vi "Features_SpecPage.vi"(10 "Spec Page Interface":T5, 11 "MetaDataObj in":refnum<class "MetaDataObj.lvclass">) -> (3 "MetaDataObj out":refnum<class "MetaDataObj.lvclass">)   [LabVIEW 2013, in "FixedChannelTBModuleDecideFeatures.lvclass"]
uses:
  FixedChannelTBModuleDecideFeatures.lvclass
  <resource>/dialog/NewProjectWizard/Spec Page Interface.ctl
  <resource>/dialog/NewProjectWizard/MetaDataObj/MetaDataObj.lvclass
  channel configuration.ctl
  <vilib>/NI/Tag Bus Module Framework/channel/channel classification.ctl
  <vilib>/NI/Tag Bus/tag/Data Type.ctl
  <resource>/dialog/NewProjectWizard/MetaDataObj/MetaDataObj.lvclass/MetaDataObj.ctl
  FixedChannelTBModuleDecideFeatures.lvclass/FixedChannelTBModuleDecideFeatures.ctl
  <resource>/dialog/NewProjectWizard/MetaDataObj/Accessors/Write Project Name.vi
  <resource>/dialog/NewProjectWizard/MetaDataObj/Accessors/Write Project Root.vi
  Write component name.vi
  Write instances allowed.vi
  <resource>/dialog/NewProjectWizard/MetaDataObj/Accessors/Write File Prefix.vi
  <vilib>/NI/Tag Bus Module Framework/channel/TBM channel.lvclass
  <vilib>/NI/Tag Bus/tag/tag descriptor.lvclass
panel:
  in  "Tab Control":T1(tab)
  in  "Channels to create":T2[](array[typedef])
  in  "Instances Allowed":i32=-1
  in  "Module Name":string
  in  "Project Root":path
  # "This script will generate a TBM with three methods in which you can add logic: User Input, User Process, and User Output. Before running this script, specify the Channel Name and Data Type for each element of data that you'd like those methods to interact with. Their are also 4 channel types to choose from.  An input channel is data generated by the input function. A processing parameter is an input to the processing function which returns processing results.  Finally an output channel is data that is passed into the output method.  \n\nThese channels can be modified later by running the User Control Module script from the LabVIEW Tools menu."
  # "Channel Name"
  # "Data Type"
  # "Channel Type"
  # "Execution Behaviors:"
  # "Number of classes allowed in a system. Default is infinite, -1. Examples: {Scaling: -1};{Scan Engine: 1}"
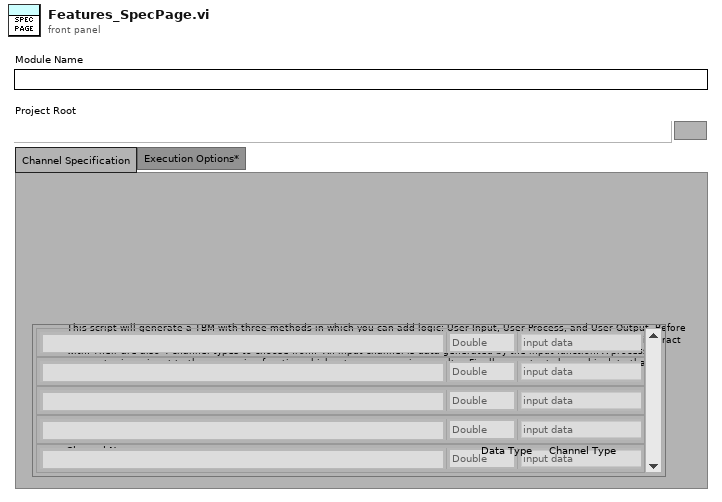
[diagram p1: front panel]
types:
  T1 = enum32{"Channel Specification", "Execution Options*"}
  T2 = typedef "FixedChannelTBModuleDecideFeatures.lvclass/channel configuration.ctl" = cluster{"Name":string, "channel classification":T3, "data type":T4}
  T3 = typedef "TBM channel.lvclass/channel classification.ctl" = enum16{"input data", "output data", "processing parameter", "processing result"}
  T4 = typedef "tag bus.lvlib/tag descriptor.lvclass/Data Type.ctl" = enum16{"Double", "Single", "I64", "I32", "I16", "I8", "U64", "U32", "U16", "U8", "Boolean", "String", "Array of Double", "Array of Single", "Array of I64", "Array of I32", "Array of I16", "Array of I8", "Array of U64", "Array of U32", "Array of U16", "Array of U8", "Array of Boolean", "Array of String"}
  T5 = typedef "Spec Page Interface.ctl" = cluster{"\"Tab Forward To\" Refnum":refnum<vi>, "\"Tab Backward To\" Refnum":refnum<vi>, "Errors":refnum<user-event>, "Quit":refnum<user-event>}
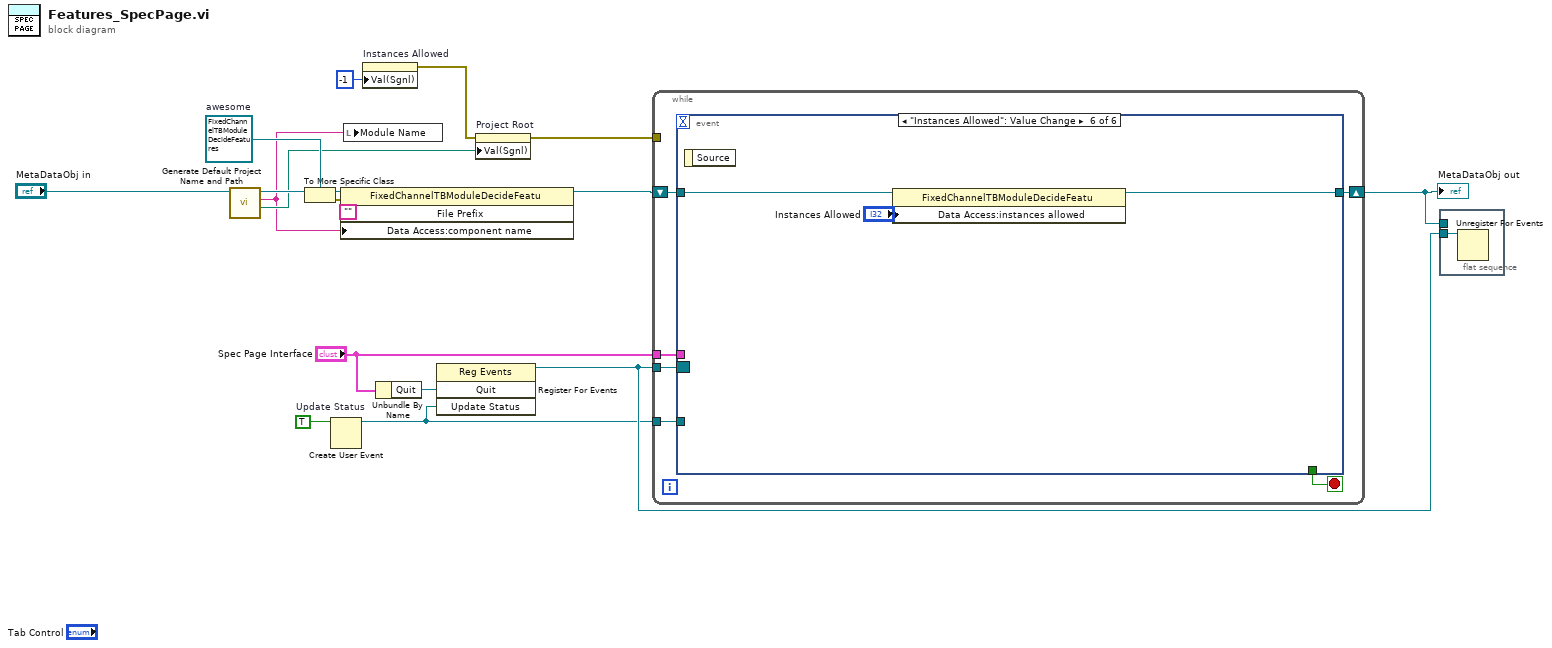
[diagram p0: block diagram]
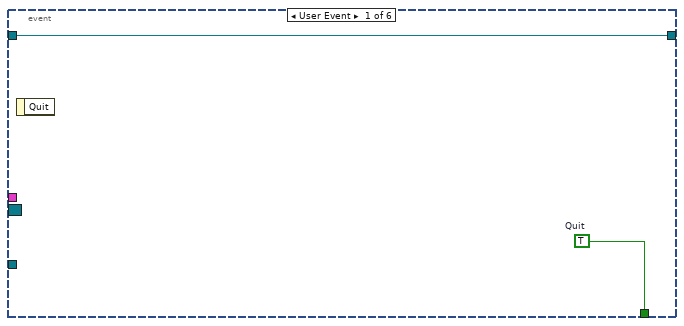
[diagram p2: hidden frame]
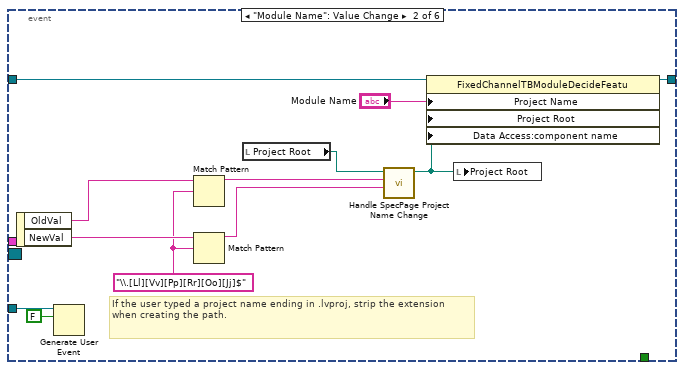
[diagram p3: hidden frame]
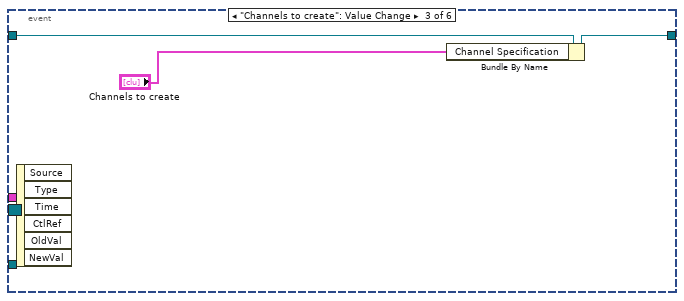
[diagram p4: hidden frame]
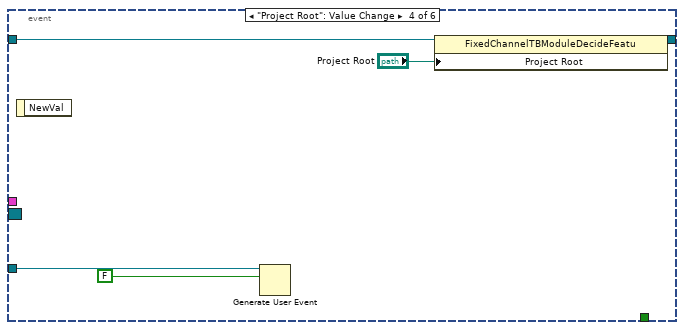
[diagram p5: hidden frame]
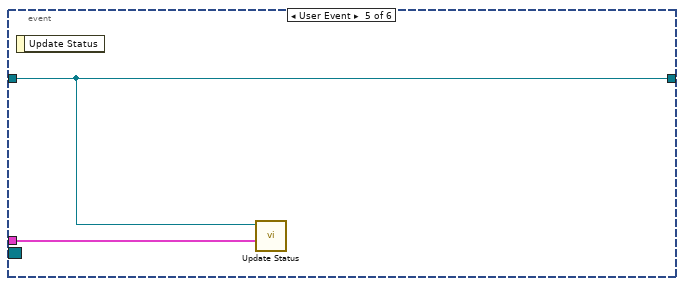
[diagram p6: hidden frame]
diagram:
  w12 = TRUE  # Update Status
  w13 = refnum<class "FixedChannelTBModuleDecideFeatures.lvclass"> refnum  # awesome
  n1 = call <resource>:"Generate Default Project Name and Path.vi"("DNL_MetaDataObj in"="MetaDataObj in") -> ("Project Root"=w5:path, "Project Name"=w3:string, "DNL_MetaDataObj out"=w6:refnum<class "MetaDataObj.lvclass">)  [unwired: 8 in]
  n2 = To More Specific Class(target class=w13, reference=w6) -> (specific class reference=w15:refnum<class "FixedChannelTBModuleDecideFeatures.lvclass">, error out=w14:errorcluster)  [unwired: 1 in]
  n3 = Create User Event(user event datatype=w12) -> (user event=w9:refnum<user-event>)  [unwired: 1 in, 1 out]
  n4 = property class="FixedChannelTBModuleDecideFeatu"(reference=w15, error in=w14, "File Prefix"="", "Data Access:component name"=w3) -> (reference out=w11:refnum<class "FixedChannelTBModuleDecideFeatures.lvclass">)  [unwired: 1 out]
  n5 = local write "Module Name"(w3) -> ()
  n6 = property on="Instances Allowed" class="DigNum (strict)"("Val(Sgnl)"=-1 ("Value (Signaling)")) -> (error out=w2:errorcluster)  [unwired: 2 in, 1 out]
  n7 = Unbundle By Name("Spec Page Interface") -> ("Quit"=w18:refnum<user-event>)
  n8 = register-events(w18, w9) -> (reference out=w17:refnum<event-registration>)  [unwired: 2 in, 1 out]
  n9 = property on="Project Root" class="Path"(error in=w2, "Val(Sgnl)"=w5) -> (error out=w10:errorcluster)  [unwired: 1 in, 1 out]
  n10 = while {
    tunnel: "Spec Page Interface" -> [w23]
    shift-right: [w21] -> w4
    shift-left: w11 -> [w20]
    tunnel: w17 -> [w22]
    tunnel: w10 -> [_]
    tunnel: w9 -> [w19]
    stop <- w24 stop-if-true
    n11 = event shown="[5] \"Instances Allowed\": Value Change" {
      selector: w22 -> [_ _ _ _ _ _]
      dyn-events: _ -> [_ _ _ _ _ _]
      timeout: _ -> [_ _ _ _ _ _]
      tunnel: w23 -> [_ _ _ _ w47 _]
      tunnel: [w26 _ _ _ _ _] -> w24
      tunnel: [w25 w38 w40 w45 w48 w50] -> w21
      tunnel: w20 -> [w25 w35 w41 w46 w48 w51]
      tunnel: w19 -> [_ w37 _ w44 _ _]
      event User Event {
        w26 = TRUE  # Quit
        n12 = event-data() -> ()  [unwired: 1 in, 1 out]
      }
      event "Module Name": Value Change {
        w30 = "\\.[Ll][Vv][Pp][Rr][Oo][Jj]$" ("regular expression")
        # "If the user typed a project name ending in .lvproj, strip the extension when creating the path."
        n13 = event-data() -> ("OldVal"=w32:string, "NewVal"=w31:string)  [unwired: 1 in]
        n14 = Generate User Event(user event=w37, event data cluster=FALSE ("Update Status")) -> ()  [unwired: 2 in, 2 out]
        n15 = Match Pattern(string=w32, regular expression=w30) -> (before substring=w29:string)  [unwired: 1 in, 3 out]
        n16 = Match Pattern(string=w31, regular expression=w30) -> (before substring=w28:string)  [unwired: 1 in, 3 out]
        n17 = local read "Project Root"() -> (w34:path)
        n18 = call <resource>:"Handle SpecPage Project Name Change.vi"("Project Name New Value"=w28, "Project Name Old Value"=w29, "Project Root in"=w34) -> ("Project Root out"=w33:path)  [unwired: 8 in]
        n19 = property class="FixedChannelTBModuleDecideFeatu"(reference=w35, "Project Name"="Module Name", "Project Root"=w33, "Data Access:component name"="Module Name") -> (reference out=w38:refnum<class "FixedChannelTBModuleDecideFeatures.lvclass">)  [unwired: 1 in, 1 out]
        n20 = local write "Project Root"(w33) -> ()
      }
      event "Channels to create": Value Change {
        n21 = event-data() -> ()  [unwired: 1 in, 6 out]
        n22 = Bundle By Name(cluster=w41, "Channel Specification"="Channels to create") -> (w40:refnum<class "FixedChannelTBModuleDecideFeatures.lvclass">)
      }
      event "Project Root": Value Change {
        n23 = event-data() -> ()  [unwired: 1 in, 1 out]
        n24 = Generate User Event(user event=w44, event data cluster=FALSE ("Update Status")) -> ()  [unwired: 2 in, 2 out]
        n25 = property class="FixedChannelTBModuleDecideFeatu"(reference=w46, "Project Root"="Project Root") -> (reference out=w45:refnum<class "FixedChannelTBModuleDecideFeatures.lvclass">)  [unwired: 1 in, 1 out]
      }
      event User Event {
        n26 = event-data() -> ()  [unwired: 1 in, 1 out]
        n27 = call "Update Status.vi"("Spec Page Interface"=w47, "TwoTasksMetaDataObj in"=w48) -> ()  [unwired: 10 in]
      }
      event "Instances Allowed": Value Change {
        n28 = event-data() -> ()  [unwired: 1 in, 1 out]
        n29 = property class="FixedChannelTBModuleDecideFeatu"(reference=w51, "Data Access:instances allowed"="Instances Allowed") -> (reference out=w50:refnum<class "FixedChannelTBModuleDecideFeatures.lvclass">)  [unwired: 1 in, 1 out]
      }
    }
  }
  "MetaDataObj out" <- w4
  n30 = flat-sequence {
    tunnel: w17 -> [w52]
    tunnel: w4 -> [_]
    frame #0 {
      n31 = Unregister For Events(event registration refnum=w52) -> ()  [unwired: 1 in, 1 out]
    }
  }
